vi "BarcodeScanner.vi"   [LabVIEW 2016]
uses:
  <vilib>/NXT/Dual Mode Library/Waits/Wait_EV3_Color_Reflected_Less.vi
  <vilib>/NXT/NXTIO Xnodes/NXTIONodeSubVIs/LEGOMoveAllMotorsDistance.vi
  <vilib>/NXT/Dual Mode Library/Sensors/EV3_Color_Reflect.vi
  <vilib>/NXT/Dual Mode Library/Display/drawText.vi
  <vilib>/NXT/Dual Mode Library/Sound/PlayF.vi
  <vilib>/NXT/NXTIO Xnodes/NXTIONodeSubVIs/LEGOMoveAllMotors.vi
  <vilib>/NXT/NXTIO Xnodes/NXTIOXNode/NXTIO.xnode
  <vilib>/NXT/Subs/LVHSConnector.ctl
  <vilib>/NXT/LegoClasses/BrickReference/BrickReference.lvclass
types:
  T1 = typedef "LVHSConnector.ctl" = refnum<class "BrickReference.lvclass">
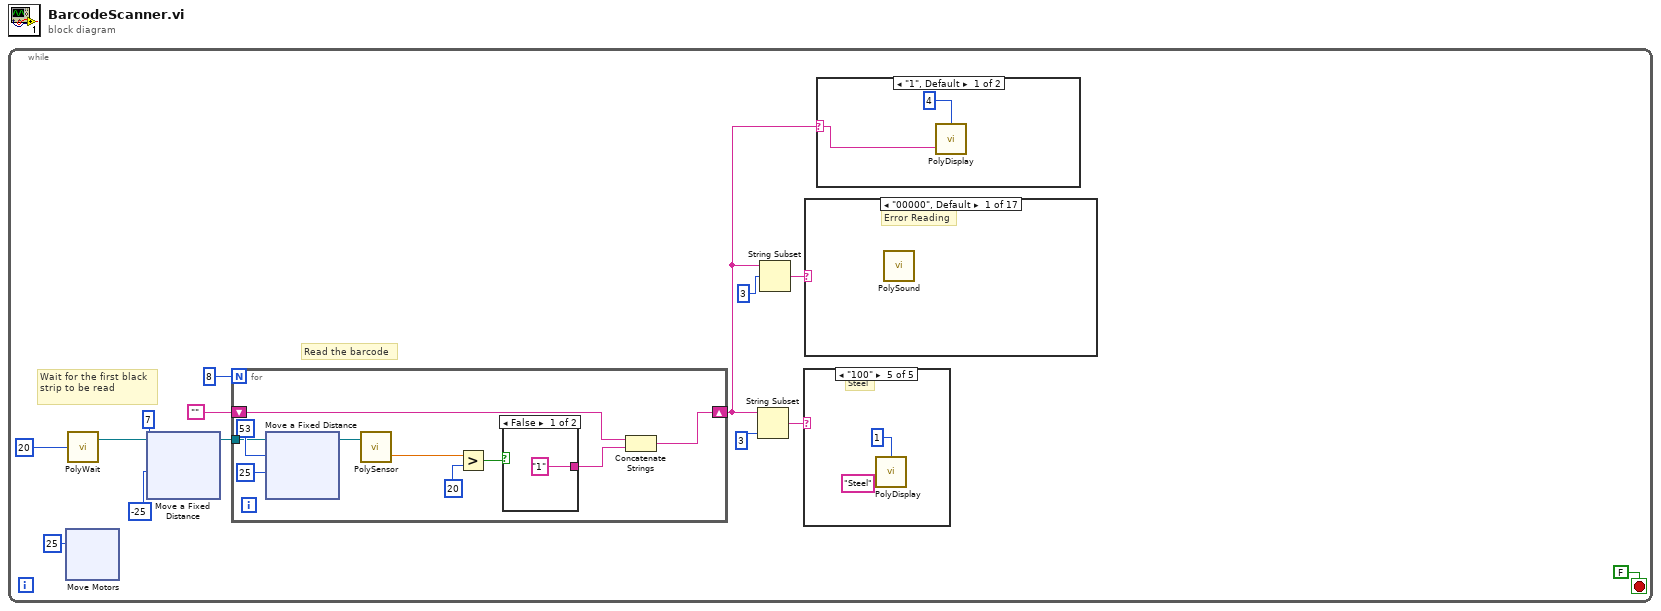
[diagram p0: block diagram]
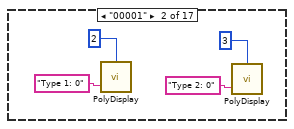
[diagram p3: hidden frame]
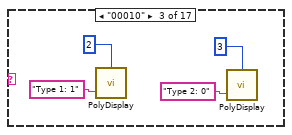
[diagram p4: hidden frame]
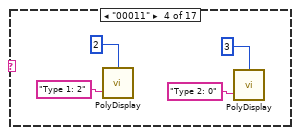
[diagram p5: hidden frame]
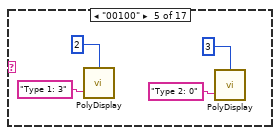
[diagram p6: hidden frame]
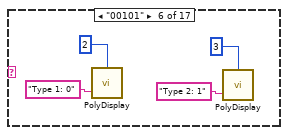
[diagram p7: hidden frame]
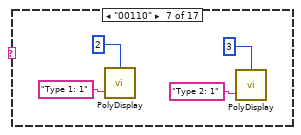
[diagram p8: hidden frame]
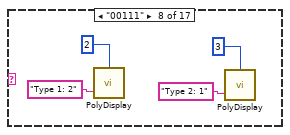
[diagram p9: hidden frame]
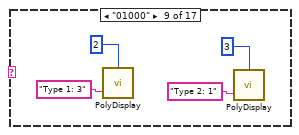
[diagram p10: hidden frame]
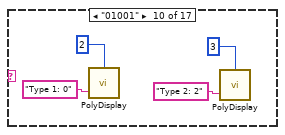
[diagram p11: hidden frame]
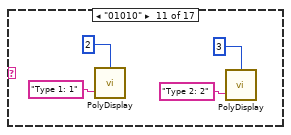
[diagram p12: hidden frame]
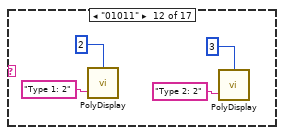
[diagram p13: hidden frame]
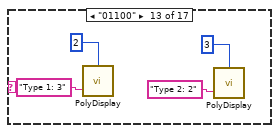
[diagram p14: hidden frame]
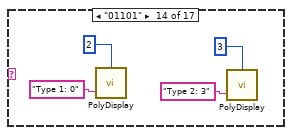
[diagram p15: hidden frame]
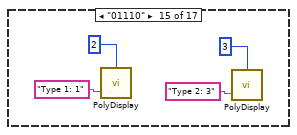
[diagram p16: hidden frame]
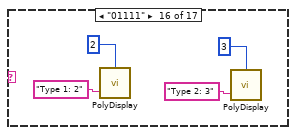
[diagram p17: hidden frame]
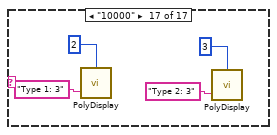
[diagram p18: hidden frame]
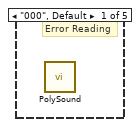
[diagram p19: hidden frame]
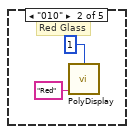
[diagram p20: hidden frame]
diagram:
  n1 = while {
    stop <- FALSE stop-if-true
    # "Read the barcode"
    # "Wait for the first black strip to be read"
    n2 = xnode "Move Motors"("Power/Speed 1"=25) -> ()  [unwired: 2 in, 1 out]
    n3 = call-poly <vilib>:"PolyWait.vi"("Scaled Value (30)"=20) -> ("NXT/EV3"=w6:T1)  [unwired: 3 in]
    n4 = xnode "Move a Fixed Distance"("Speed 1"=-25, "Distance 1"=7, "NXT/EV3"=w6) -> ("NXT/EV3"=w9:T1)  [unwired: 1 in]
    n5 = for {
      N: 8 -> [_]
      shift-right: [w112] -> w1
      shift-left: "" -> [w113]
      tunnel: w9 -> [w105]
      n6 = xnode "Move a Fixed Distance"("Speed 1"=25, "Distance 1"=53, "NXT/EV3"=w105) -> ("NXT/EV3"=w109:T1)  [unwired: 1 in]
      n7 = call-poly <vilib>:"PolySensor.vi"("NXT/EV3"=w109) -> ("Scaled Value"=w108:sgl)  [unwired: 2 in, 1 out]
      n8 = Greater?(x=w108, y=20) -> (0:w104:bool)
      n9 = case shown="False" w104 {
        tunnel: ["1" "0"] -> w106
        frame False {
        }
        frame True {
        }
      }
      n10 = Concatenate Strings(w113, w106) -> (w112:string)
    }
    n11 = String Subset(string=w1, length (rest)=3) -> (substring=w11:string)  [unwired: 1 in]
    n12 = String Subset(string=w1, offset (0)=3) -> (substring=w2:string)  [unwired: 1 in]
    n13 = case shown="\"100\"" w11 {
      frame "000", Default {
        # "Error Reading"
        n14 = call-poly <vilib>:"PolySound.vi"() -> ()  [unwired: 4 in, 1 out]
      }
      frame "010" {
        # "Red Glass"
        n15 = call-poly <vilib>:"PolyDisplay.vi"("Text"="Red", "Line"=1) -> ()  [unwired: 2 in, 1 out]
      }
      frame "001" {
        # "White Glass"
        n16 = call-poly <vilib>:"PolyDisplay.vi"("Text"="White", "Line"=1) -> ()  [unwired: 2 in, 1 out]
      }
      frame "011" {
        # "Blue Glass"
        n17 = call-poly <vilib>:"PolyDisplay.vi"("Text"="Blue", "Line"=1) -> ()  [unwired: 2 in, 1 out]
      }
      frame "100" {
        # "Steel"
        n18 = call-poly <vilib>:"PolyDisplay.vi"("Text"="Steel", "Line"=1) -> ()  [unwired: 2 in, 1 out]
      }
    }
    n19 = case shown="\"00000\", Default" w2 {
      frame "00000", Default {
        # "Error Reading"
        n20 = call-poly <vilib>:"PolySound.vi"() -> ()  [unwired: 4 in, 1 out]
      }
      frame "00001" {
        n21 = call-poly <vilib>:"PolyDisplay.vi"("Text"="Type 1: 0", "Line"=2) -> ()  [unwired: 2 in, 1 out]
        n22 = call-poly <vilib>:"PolyDisplay.vi"("Text"="Type 2: 0", "Line"=3) -> ()  [unwired: 2 in, 1 out]
      }
      frame "00010" {
        n23 = call-poly <vilib>:"PolyDisplay.vi"("Text"="Type 1: 1", "Line"=2) -> ()  [unwired: 2 in, 1 out]
        n24 = call-poly <vilib>:"PolyDisplay.vi"("Text"="Type 2: 0", "Line"=3) -> ()  [unwired: 2 in, 1 out]
      }
      frame "00011" {
        n25 = call-poly <vilib>:"PolyDisplay.vi"("Text"="Type 1: 2", "Line"=2) -> ()  [unwired: 2 in, 1 out]
        n26 = call-poly <vilib>:"PolyDisplay.vi"("Text"="Type 2: 0", "Line"=3) -> ()  [unwired: 2 in, 1 out]
      }
      frame "00100" {
        n27 = call-poly <vilib>:"PolyDisplay.vi"("Text"="Type 1: 3", "Line"=2) -> ()  [unwired: 2 in, 1 out]
        n28 = call-poly <vilib>:"PolyDisplay.vi"("Text"="Type 2: 0", "Line"=3) -> ()  [unwired: 2 in, 1 out]
      }
      frame "00101" {
        n29 = call-poly <vilib>:"PolyDisplay.vi"("Text"="Type 1: 0", "Line"=2) -> ()  [unwired: 2 in, 1 out]
        n30 = call-poly <vilib>:"PolyDisplay.vi"("Text"="Type 2: 1", "Line"=3) -> ()  [unwired: 2 in, 1 out]
      }
      frame "00110" {
        n31 = call-poly <vilib>:"PolyDisplay.vi"("Text"="Type 1: 1", "Line"=2) -> ()  [unwired: 2 in, 1 out]
        n32 = call-poly <vilib>:"PolyDisplay.vi"("Text"="Type 2: 1", "Line"=3) -> ()  [unwired: 2 in, 1 out]
      }
      frame "00111" {
        n33 = call-poly <vilib>:"PolyDisplay.vi"("Text"="Type 1: 2", "Line"=2) -> ()  [unwired: 2 in, 1 out]
        n34 = call-poly <vilib>:"PolyDisplay.vi"("Text"="Type 2: 1", "Line"=3) -> ()  [unwired: 2 in, 1 out]
      }
      frame "01000" {
        n35 = call-poly <vilib>:"PolyDisplay.vi"("Text"="Type 1: 3", "Line"=2) -> ()  [unwired: 2 in, 1 out]
        n36 = call-poly <vilib>:"PolyDisplay.vi"("Text"="Type 2: 1", "Line"=3) -> ()  [unwired: 2 in, 1 out]
      }
      frame "01001" {
        n37 = call-poly <vilib>:"PolyDisplay.vi"("Text"="Type 1: 0", "Line"=2) -> ()  [unwired: 2 in, 1 out]
        n38 = call-poly <vilib>:"PolyDisplay.vi"("Text"="Type 2: 2", "Line"=3) -> ()  [unwired: 2 in, 1 out]
      }
      frame "01010" {
        n39 = call-poly <vilib>:"PolyDisplay.vi"("Text"="Type 1: 1", "Line"=2) -> ()  [unwired: 2 in, 1 out]
        n40 = call-poly <vilib>:"PolyDisplay.vi"("Text"="Type 2: 2", "Line"=3) -> ()  [unwired: 2 in, 1 out]
      }
      frame "01011" {
        n41 = call-poly <vilib>:"PolyDisplay.vi"("Text"="Type 1: 2", "Line"=2) -> ()  [unwired: 2 in, 1 out]
        n42 = call-poly <vilib>:"PolyDisplay.vi"("Text"="Type 2: 2", "Line"=3) -> ()  [unwired: 2 in, 1 out]
      }
      frame "01100" {
        n43 = call-poly <vilib>:"PolyDisplay.vi"("Text"="Type 1: 3", "Line"=2) -> ()  [unwired: 2 in, 1 out]
        n44 = call-poly <vilib>:"PolyDisplay.vi"("Text"="Type 2: 2", "Line"=3) -> ()  [unwired: 2 in, 1 out]
      }
      frame "01101" {
        n45 = call-poly <vilib>:"PolyDisplay.vi"("Text"="Type 1: 0", "Line"=2) -> ()  [unwired: 2 in, 1 out]
        n46 = call-poly <vilib>:"PolyDisplay.vi"("Text"="Type 2: 3", "Line"=3) -> ()  [unwired: 2 in, 1 out]
      }
      frame "01110" {
        n47 = call-poly <vilib>:"PolyDisplay.vi"("Text"="Type 1: 1", "Line"=2) -> ()  [unwired: 2 in, 1 out]
        n48 = call-poly <vilib>:"PolyDisplay.vi"("Text"="Type 2: 3", "Line"=3) -> ()  [unwired: 2 in, 1 out]
      }
      frame "01111" {
        n49 = call-poly <vilib>:"PolyDisplay.vi"("Text"="Type 1: 2", "Line"=2) -> ()  [unwired: 2 in, 1 out]
        n50 = call-poly <vilib>:"PolyDisplay.vi"("Text"="Type 2: 3", "Line"=3) -> ()  [unwired: 2 in, 1 out]
      }
      frame "10000" {
        n51 = call-poly <vilib>:"PolyDisplay.vi"("Text"="Type 1: 3", "Line"=2) -> ()  [unwired: 2 in, 1 out]
        n52 = call-poly <vilib>:"PolyDisplay.vi"("Text"="Type 2: 3", "Line"=3) -> ()  [unwired: 2 in, 1 out]
      }
    }
    n53 = case shown="\"1\", Default" w1 {
      selector: w1 -> [w15 _]
      frame "1", Default {
        n54 = call-poly <vilib>:"PolyDisplay.vi"("Text"=w15, "Line"=4) -> ()  [unwired: 2 in, 1 out]
      }
      frame "True2" {
      }
    }
  }
